vi "PLC Shutdown.vi"(8 "error in":errorcluster, 11 "Modbus master in":refnum<class "Modbus Master.lvclass">) -> (0 "error out":errorcluster, 3 "Modbus master out":refnum<class "Modbus Master.lvclass">)   [LabVIEW 2014, in "Main Libraryv2.lvlib"]
uses:
  Control/Main Libraryv2.lvlib
  <vilib>/NI/Modbus Library/API/Master/Modbus Master.lvclass
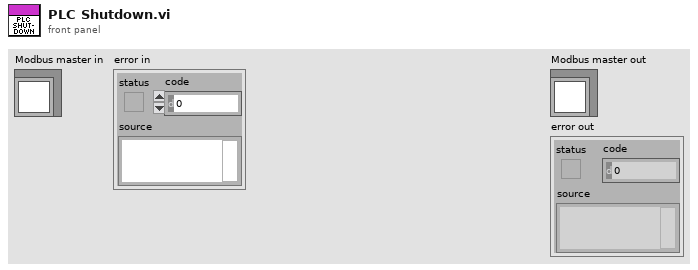
[diagram p1: front panel]
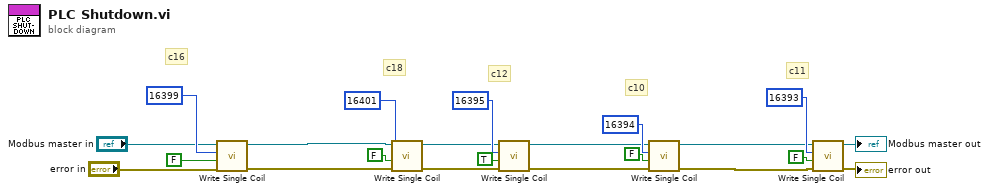
[diagram p0: block diagram]
diagram:
  # "c16"
  # "c11"
  # "c10"
  # "c12"
  # "c18"
  n1 = call-dynamic "Write Single Coil.vi"("error in"="error in", "coil to write"=FALSE, "address"=u16 16399, "Modbus master in"="Modbus master in") -> ("error out"=w9:errorcluster, "Modbus master out"=w10:refnum<class "Modbus Master.lvclass">)  [unwired: 6 in]
  n2 = call-dynamic "Write Single Coil.vi"("error in"=w9, "coil to write"=FALSE, "address"=u16 16401, "Modbus master in"=w10) -> ("error out"=w7:errorcluster, "Modbus master out"=w8:refnum<class "Modbus Master.lvclass">)  [unwired: 6 in]
  n3 = call-dynamic "Write Single Coil.vi"("error in"=w7, "coil to write"=TRUE, "address"=u16 16395, "Modbus master in"=w8) -> ("error out"=w5:errorcluster, "Modbus master out"=w6:refnum<class "Modbus Master.lvclass">)  [unwired: 6 in]
  n4 = call-dynamic "Write Single Coil.vi"("error in"=w5, "coil to write"=FALSE, "address"=u16 16394, "Modbus master in"=w6) -> ("error out"=w3:errorcluster, "Modbus master out"=w4:refnum<class "Modbus Master.lvclass">)  [unwired: 6 in]
  n5 = call-dynamic "Write Single Coil.vi"("error in"=w3, "coil to write"=FALSE, "address"=u16 16393, "Modbus master in"=w4) -> ("error out"=→"error out":errorcluster, "Modbus master out"=→"Modbus master out":refnum<class "Modbus Master.lvclass">)  [unwired: 6 in]
